vi "HAL process.vi"   [LabVIEW 2016]
uses:
  <vilib>/Plasmionique/MB Master/MB_Master/MB_Master.lvclass
  PLC/PLC.lvlib
types:
  T1 = cluster{"水样测试量程模式":enum16{"H", "L", "AUTO"}, "空白核查量程模式":enum16{"H", "L", "AUTO"}, "跨度核查量程模式":enum16{"H", "L", "AUTO"}, "加标回收量程模式":enum16{"H", "L", "AUTO"}}
  T2 = cluster{"因子编码":u32, "单位":u16, "标样参考值":sgl, "水样数据时间":timestamp, "水样实测值":sgl, "水样数据标识":string, "标样数据时间":timestamp, "标样实测值":sgl, "标样数据标识":string, "空白数据时间":timestamp, "空白实测值":sgl, "空白数据标识":string, "零点核查数据时间":timestamp, "零点核查实测值":sgl, "零点核查数据标识":string, "跨度核查数据时间":timestamp, "跨度核查实测值":sgl, "跨度核查数据标识":string, "加标回收数据时间":timestamp, "加标回收实测值":sgl, "加标回收数据标识":string, "平行样数据时间":timestamp, "平行样实测值":sgl, "平行样数据标识":string}
  T3 = cluster{"SYSTEM Interface":cluster{"运行模式":enum16{"维护模式", "常规模式", "应急模式", "质控模式"}, "站点类型":enum16{"一体站", "固定站"}, "CODMn类型":enum16{"PLC版", "单片机版"}}, "Pump Interface":cluster{"Pump MB session in":refnum<class "MB_Master.lvclass">}, "NH3N Interface":cluster{"NH3N session in":refnum<class "MB_Master.lvclass">, "氨氮自动测试量程配置":cluster{"水样测试量程模式":enum16{"H", "L", "AUTO"}, "空白核查量程模式":enum16{"H", "L", "AUTO"}, "跨度核查量程模式":enum16{"H", "L", "AUTO"}, "加标回收量程模式":enum16{"H", "L", "AUTO"}}}, "TP Interface":cluster{"TP MB session in":refnum<class "MB_Master.lvclass">, "总磷自动测试量程配置":cluster{"水样测试量程模式":enum16{"H", "L", "AUTO"}, "空白核查量程模式":enum16{"H", "L", "AUTO"}, "跨度核查量程模式":enum16{"H", "L", "AUTO"}, "加标回收量程模式":enum16{"H", "L", "AUTO"}}}, "TN Interface":cluster{"TN MB session in":refnum<class "MB_Master.lvclass">, "总氮自动测试量程配置":cluster{"水样测试量程模式":enum16{"H", "L", "AUTO"}, "空白核查量程模式":enum16{"H", "L", "AUTO"}, "跨度核查量程模式":enum16{"H", "L", "AUTO"}, "加标回收量程模式":enum16{"H", "L", "AUTO"}}}, "CODMn Interface":cluster{"CODMn MB session in":refnum<class "MB_Master.lvclass">, "CODMn自动测试量程配置":cluster{"水样测试量程模式":enum16{"H", "L", "AUTO"}, "空白核查量程模式":enum16{"H", "L", "AUTO"}, "跨度核查量程模式":enum16{"H", "L", "AUTO"}, "加标回收量程模式":enum16{"H", "L", "AUTO"}}}, "CODCr Interface":cluster{"CODCr MB session in":refnum<class "MB_Master.lvclass">, "CODCr自动测试量程配置":cluster{"水样测试量程模式":enum16{"H", "L", "AUTO"}, "空白核查量程模式":enum16{"H", "L", "AUTO"}, "跨度核查量程模式":enum16{"H", "L", "AUTO"}, "加标回收量程模式":enum16{"H", "L", "AUTO"}}}, "PLC_CODMn Interface":cluster{"PLC版_CODMn状态":u16, "PLC版_CODMn测量数据区":cluster{"因子编码":u32, "单位":u16, "标样参考值":sgl, "水样数据时间":timestamp, "水样实测值":sgl, "水样数据标识":string, "标样数据时间":timestamp, "标样实测值":sgl, "标样数据标识":string, "空白数据时间":timestamp, "空白实测值":sgl, "空白数据标识":string, "零点核查数据时间":timestamp, "零点核查实测值":sgl, "零点核查数据标识":string, "跨度核查数据时间":timestamp, "跨度核查实测值":sgl, "跨度核查数据标识":string, "加标回收数据时间":timestamp, "加标回收实测值":sgl, "加标回收数据标识":string, "平行样数据时间":timestamp, "平行样实测值":sgl, "平行样数据标识":string}}}
  T4 = cluster{"水样测试量程模式":enum16{"H", "L", "AUTO"}, "空白核查量程模式":enum16{"H", "L", "AUTO"}, "跨度核查量程模式":enum16{"H", "L", "AUTO"}, "加标回收量程模式":enum16{"H", "L", "AUTO"}, "标样核查量程模式":enum16{"H", "L", "AUTO"}}
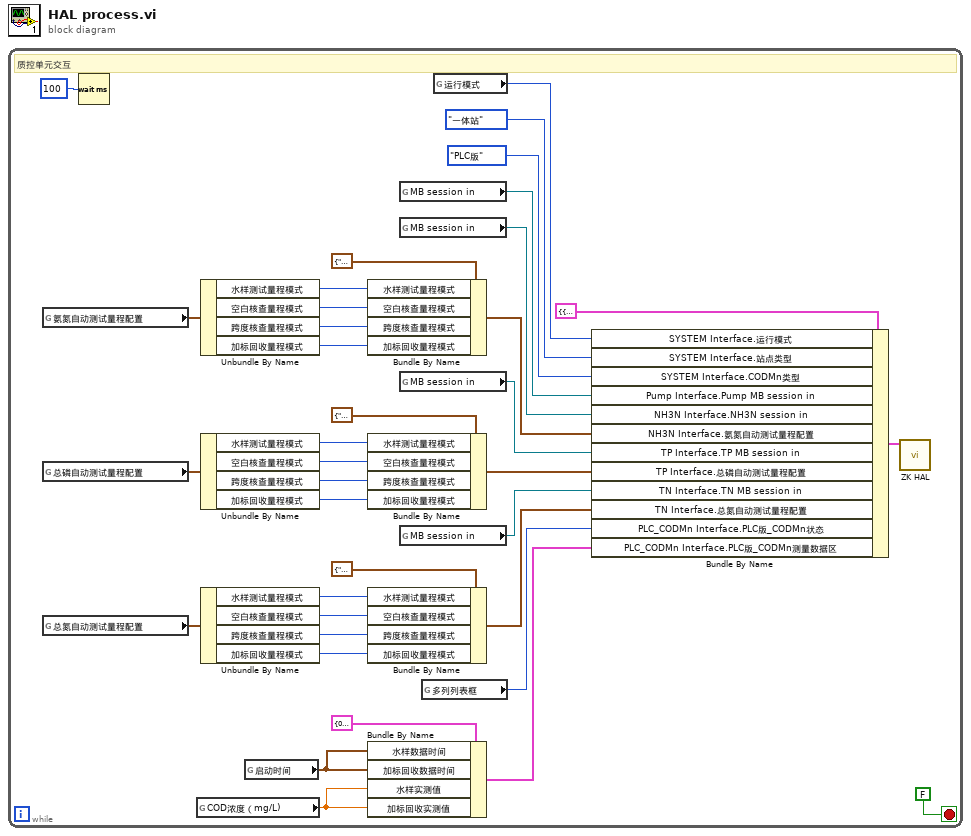
[diagram p0: block diagram]
diagram:
  n1 = while {
    stop <- FALSE stop-if-true
    # "质控单元交互"
    n2 = global read "总磷总氮断电保存全局变量.vi" "氨氮自动测试量程配置"() -> (w20:T4)
    n3 = global read "总磷总氮断电保存全局变量.vi" "总磷自动测试量程配置"() -> (w8:T4)
    n4 = global read "总磷总氮断电保存全局变量.vi" "总氮自动测试量程配置"() -> (w2:T4)
    n5 = Wait (ms)(milliseconds to wait=u32 100 ("等待时间（毫秒）")) -> ()  [unwired: 1 out]
    n6 = global read "COD浓度全局变量.vi" "COD浓度（mg/L)"() -> (w25:dbl)
    n7 = Unbundle By Name(w20) -> ("水样测试量程模式"=w18:enum16{"H", "L", "AUTO"}, "空白核查量程模式"=w17:enum16{"H", "L", "AUTO"}, "跨度核查量程模式"=w16:enum16{"H", "L", "AUTO"}, "加标回收量程模式"=w15:enum16{"H", "L", "AUTO"})
    n8 = Unbundle By Name(w8) -> ("水样测试量程模式"=w11:enum16{"H", "L", "AUTO"}, "空白核查量程模式"=w12:enum16{"H", "L", "AUTO"}, "跨度核查量程模式"=w13:enum16{"H", "L", "AUTO"}, "加标回收量程模式"=w14:enum16{"H", "L", "AUTO"})
    n9 = Unbundle By Name(w2) -> ("水样测试量程模式"=w6:enum16{"H", "L", "AUTO"}, "空白核查量程模式"=w5:enum16{"H", "L", "AUTO"}, "跨度核查量程模式"=w4:enum16{"H", "L", "AUTO"}, "加标回收量程模式"=w3:enum16{"H", "L", "AUTO"})
    n10 = global read "CODMn断电保存全局变量.vi" "启动时间"() -> (w22:timestamp)
    n11 = Bundle By Name(cluster=T1 {"水样测试量程模式"=enum."H", "空白核查量程模式"=enum."H", "跨度核查量程模式"=enum."H", "加标回收量程模式"=enum."H"} ("NH3N Interface.氨氮自动测试量程配置"), "水样测试量程模式"=w18, "空白核查量程模式"=w17, "跨度核查量程模式"=w16, "加标回收量程模式"=w15) -> (w19:T1)
    n12 = Bundle By Name(cluster=T1 {"水样测试量程模式"=enum."H", "空白核查量程模式"=enum."H", "跨度核查量程模式"=enum."H", "加标回收量程模式"=enum."H"} ("NH3N Interface.氨氮自动测试量程配置"), "水样测试量程模式"=w11, "空白核查量程模式"=w12, "跨度核查量程模式"=w13, "加标回收量程模式"=w14) -> (w9:T1)
    n13 = Bundle By Name(cluster=T1 {"水样测试量程模式"=enum."H", "空白核查量程模式"=enum."H", "跨度核查量程模式"=enum."H", "加标回收量程模式"=enum."H"} ("NH3N Interface.氨氮自动测试量程配置"), "水样测试量程模式"=w6, "空白核查量程模式"=w5, "跨度核查量程模式"=w4, "加标回收量程模式"=w3) -> (w1:T1)
    n14 = Bundle By Name(cluster=T2 {"因子编码"=0, "单位"=0, "标样参考值"=0.0, "水样数据时间"=timestamp(0 s since 1904-01-01), "水样实测值"=0.0, "水样数据标识"="", "标样数据时间"=timestamp(0 s since 1904-01-01), "标样实测值"=0.0, "标样数据标识"="", "空白数据时间"=timestamp(0 s since 1904-01-01), "空白实测值"=0.0, "空白数据标识"="", "零点核查数据时间"=timestamp(0 s since 1904-01-01), "零点核查实测值"=0.0, "零点核查数据标识"="", "跨度核查数据时间"=timestamp(0 s since 1904-01-01), "跨度核查实测值"=0.0, "跨度核查数据标识"="", "加标回收数据时间"=timestamp(0 s since 1904-01-01), "加标回收实测值"=0.0, "加标回收数据标识"="", "平行样数据时间"=timestamp(0 s since 1904-01-01), "平行样实测值"=0.0, "平行样数据标识"=""} ("PLC_CODMn Interface.PLC版_CODMn测量数据区"), "水样数据时间"=w22, "加标回收数据时间"=w22, "水样实测值"=w25, "加标回收实测值"=w25) -> (w23:T2)
    n15 = global read "采配水全局变量.vi" "MB session in"() -> (w30:refnum<class "MB_Master.lvclass">)
    n16 = global read "VAR总磷总氮全局变量.vi" "MB session in"() -> (w29:refnum<class "MB_Master.lvclass">)
    n17 = global read "VAR总磷总氮全局变量.vi" "MB session in"() -> (w28:refnum<class "MB_Master.lvclass">)
    n18 = global read "VAR总磷总氮全局变量.vi" "MB session in"() -> (w27:refnum<class "MB_Master.lvclass">)
    n19 = global read "运行时序全局变量.vi" "多列列表框"() -> (w26:i32)
    n20 = global read "系统设置全局变量.vi" "运行模式"() -> (w31:enum16{"维护模式", "常规模式", "应急模式", "质控模式"})
    n21 = Bundle By Name(cluster=T3 {"SYSTEM Interface"={"运行模式"=enum."维护模式", "站点类型"=enum."一体站", "CODMn类型"=enum."PLC版"}, "Pump Interface"={"Pump MB session in"=refnum}, "NH3N Interface"={"NH3N session in"=refnum, "氨氮自动测试量程配置"={"水样测试量程模式"=enum."AUTO", "空白核查量程模式"=enum."AUTO", "跨度核查量程模式"=enum."AUTO", "加标回收量程模式"=enum."AUTO"}}, "TP Interface"={"TP MB session in"=refnum, "总磷自动测试量程配置"={"水样测试量程模式"=enum."AUTO", "空白核查量程模式"=enum."AUTO", "跨度核查量程模式"=enum."AUTO", "加标回收量程模式"=enum."AUTO"}}, "TN Interface"={"TN MB session in"=refnum, "总氮自动测试量程配置"={"水样测试量程模式"=enum."AUTO", "空白核查量程模式"=enum."AUTO", "跨度核查量程模式"=enum."AUTO", "加标回收量程模式"=enum."AUTO"}}, "CODMn Interface"={"CODMn MB session in"=refnum, "CODMn自动测试量程配置"={"水样测试量程模式"=enum."AUTO", "空白核查量程模式"=enum."AUTO", "跨度核查量程模式"=enum."AUTO", "加标回收量程模式"=enum."AUTO"}}, "CODCr Interface"={"CODCr MB session in"=refnum, "CODCr自动测试量程配置"={"水样测试量程模式"=enum."AUTO", "空白核查量程模式"=enum."AUTO", "跨度核查量程模式"=enum."AUTO", "加标回收量程模式"=enum."AUTO"}}, "PLC_CODMn Interface"={"PLC版_CODMn状态"=0, "PLC版_CODMn测量数据区"={"因子编码"=0, "单位"=0, "标样参考值"=0.0, "水样数据时间"=timestamp(0 s since 1904-01-01), "水样实测值"=0.0, "水样数据标识"="", "标样数据时间"=timestamp(0 s since 1904-01-01), "标样实测值"=0.0, "标样数据标识"="", "空白数据时间"=timestamp(0 s since 1904-01-01), "空白实测值"=0.0, "空白数据标识"="", "零点核查数据时间"=timestamp(0 s since 1904-01-01), "零点核查实测值"=0.0, "零点核查数据标识"="", "跨度核查数据时间"=timestamp(0 s since 1904-01-01), "跨度核查实测值"=0.0, "跨度核查数据标识"="", "加标回收数据时间"=timestamp(0 s since 1904-01-01), "加标回收实测值"=0.0, "加标回收数据标识"="", "平行样数据时间"=timestamp(0 s since 1904-01-01), "平行样实测值"=0.0, "平行样数据标识"=""}}} ("Interface"), "SYSTEM Interface.运行模式"=w31, "SYSTEM Interface.站点类型"=enum16{"一体站", "固定站"}."一体站", "SYSTEM Interface.CODMn类型"=enum16{"PLC版", "单片机版"}."PLC版", "Pump Interface.Pump MB session in"=w30, "NH3N Interface.NH3N session in"=w29, "NH3N Interface.氨氮自动测试量程配置"=w19, "TP Interface.TP MB session in"=w28, "TP Interface.总磷自动测试量程配置"=w9, "TN Interface.TN MB session in"=w27, "TN Interface.总氮自动测试量程配置"=w1, "PLC_CODMn Interface.PLC版_CODMn状态"=w26, "PLC_CODMn Interface.PLC版_CODMn测量数据区"=w23) -> (w34:T3)
    n22 = call "ZK HAL.vi"("Interface"=w34) -> ()  [unwired: 11 in]
  }
